vi "Get Accessibility.vi"(8 "error in (no error)":errorcluster, 11 "SMO":refnum<class "SMO.lvclass">) -> (0 "error out":errorcluster, 2 "Accessibility":T1, 3 "SMO out":refnum<class "SMO.lvclass">)   [LabVIEW 2013, in "SMO.lvclass"]
uses:
  SMO.lvclass
  Typedefs/Accessibility--Cluster.ctl
  Typedefs/Reserve State--Enum.ctl
  SMO.lvclass/SMO.ctl
panel:
  # "For instructions on how to use the JKI State Machine Objects, examples and video tutorials, visit:\nhttp://jki.net/state-machine-objects/\n\nJKI State Machine Objects™\nhttp://jki.net/state-machine-objects/\nCopyright (C) 2005-2015, JKI <info@jki.net>\nALL RIGHTS RESERVED"
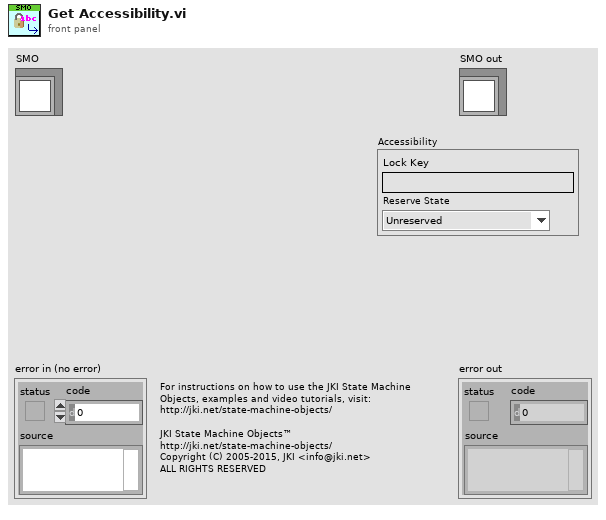
[diagram p1: front panel]
types:
  T1 = typedef "SMO.lvclass/Accessibility--Cluster.ctl" = cluster{"Lock Key":string, "Reserve State":T2}
  T2 = typedef "SMO.lvclass/Reserve State--Enum.ctl" = enum16{"Unreserved", "Reserved", "Self-locked"}
  T3 = typedef "SMO.lvclass/PrivateData--Ref.ctl" = refnum<data-value>
  T4 = typedef "SMO.lvclass/PrivateData--Cluster.ctl" = cluster{"Parent Call":T5, "Registered Processes":T6[], "Sync Notifier":refnum<notifier>, "Process Error Notifier":refnum<notifier>, "Protected Events":T7, "Public Events":T8, "SMO State":T9, "[Attributes]":variant, "Launcher Close":refnum<notifier>, "Caller Watchdog":refnum<queue>, "Accessibility":T1, "NbStaticDependencies":u32}
  T5 = typedef "SMO.lvclass/Parent Call--Enum.ctl" = enum16{"Allows parent to run", "Does not request parent to run"}
  T6 = typedef "SMO.lvclass/RegisteredProcessData--Cluster.ctl" = cluster{"Name":string, "Static VI Ref":refnum<vi>, "Running":bool, "NotifierRef":u32}
  T7 = typedef "SMO.lvclass/Protected Events.ctl" = cluster{"StopProcesses":refnum<user-event>, "AbortProcesses":refnum<user-event>, "Config Changed":refnum<user-event>, "Dependency":refnum<user-event>}
  T8 = typedef "SMO.lvclass/Public Events.ctl" = cluster{"Error":refnum<user-event>, "State":refnum<user-event>, "Reserve State":refnum<user-event>}
  T9 = typedef "SMO.lvclass/SMOState --Enum.ctl" = enum16{"unknown", "Created", "Started", "Stopped"}
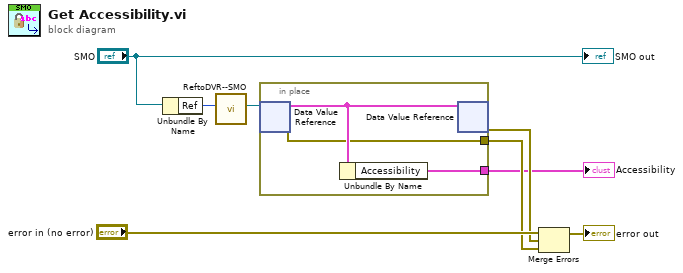
[diagram p0: block diagram]
diagram:
  n1 = Unbundle By Name("SMO") -> ("Ref"=w3:u32)
  n2 = call "ReftoDVR--SMO.vi"("Ref"=w3) -> ("Ref"=w2:T3)  [unwired: 10 in]
  n3 = in-place {
    in-place-border: [w11] -> w4
    in-place-border: [w9] -> w6
    n4 = in-place-dvr #1(w2) -> (w10:T4, w9:errorcluster)
    n5 = Unbundle By Name(w10) -> ("Accessibility"=w11:T1)
    n6 = in-place-dvr #1(w10) -> (w5:errorcluster)  [unwired: 1 out]
  }
  "Accessibility" <- w4
  n7 = Merge Errors("error in (no error)", w5, w6) -> (→"error out":errorcluster)
  "SMO out" <- "SMO"
